vi "Open Front Panel.vi"(8 "error in (no error)":errorcluster, 11 "ViewableActor in":refnum<class "ViewableActor.lvclass">) -> (0 "error out":errorcluster, 3 "ViewableActor out":refnum<class "ViewableActor.lvclass">)   [LabVIEW 2012, in "Win8uiFramework.lvlib" / "ViewableActor.lvclass"]
uses:
  ViewableActor.lvclass
  ViewableActor.lvclass/ViewableActor.ctl
  Read UI VI Ref.vi
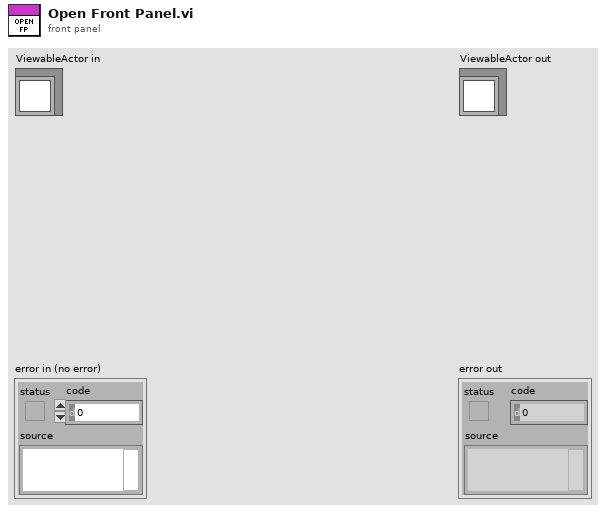
[diagram p1: front panel]
types:
  T1 = enum32{"Invalid", "Standard", "Closed", "Hidden", "Minimized", "Maximized"}
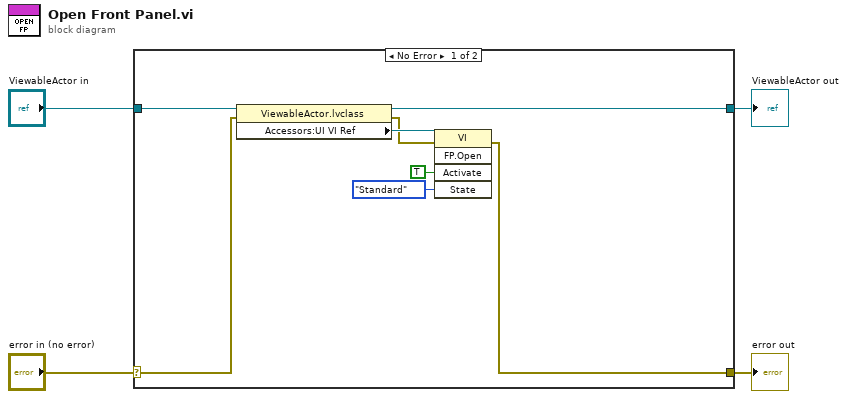
[diagram p0: block diagram]
diagram:
  n1 = case shown="No Error" "error in (no error)" {
    selector: "error in (no error)" -> [w6 w14]
    tunnel: [w5 w14] -> w3
    tunnel: [w11 w13] -> w1
    tunnel: "ViewableActor in" -> [w12 w13]
    frame No Error {
      n2 = property class="ViewableActor.lvclass"(reference=w12, error in=w6) -> (reference out=w11:refnum<class "ViewableActor.lvclass">, error out=w7:errorcluster, "Accessors:UI VI Ref"=w10:refnum<vi>)
      n3 = invoke class="VI" method="FP.Open"(reference=w10, error in=w7, "Activate"=TRUE ("Activate?"), "State"=T1."Standard") -> (error out=w5:errorcluster)  [unwired: 1 in, 4 out]
    }
    frame Error {
    }
  }
  "error out" <- w3
  "ViewableActor out" <- w1
